vi "ConnectSetVarAtt.vi"(7 "VI reference":refnum<vi>, 8 "error in (no error)":errorcluster, 10 "Terms[]":refnum<vi>[][](array[refnum])) -> (0 "error out":errorcluster)   [LabVIEW 2009, in "HGF_VisitorGenerator.lvlib"]
doc: "wire set variant attribute in visitors appendData2Variant.vi"
uses:
  HGF_VisitorGenerator.lvlib
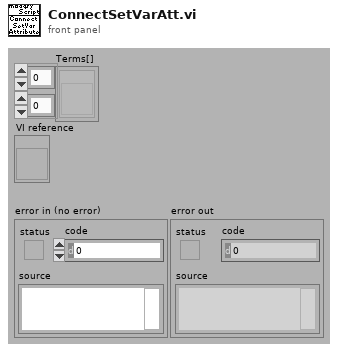
[diagram p1: front panel]
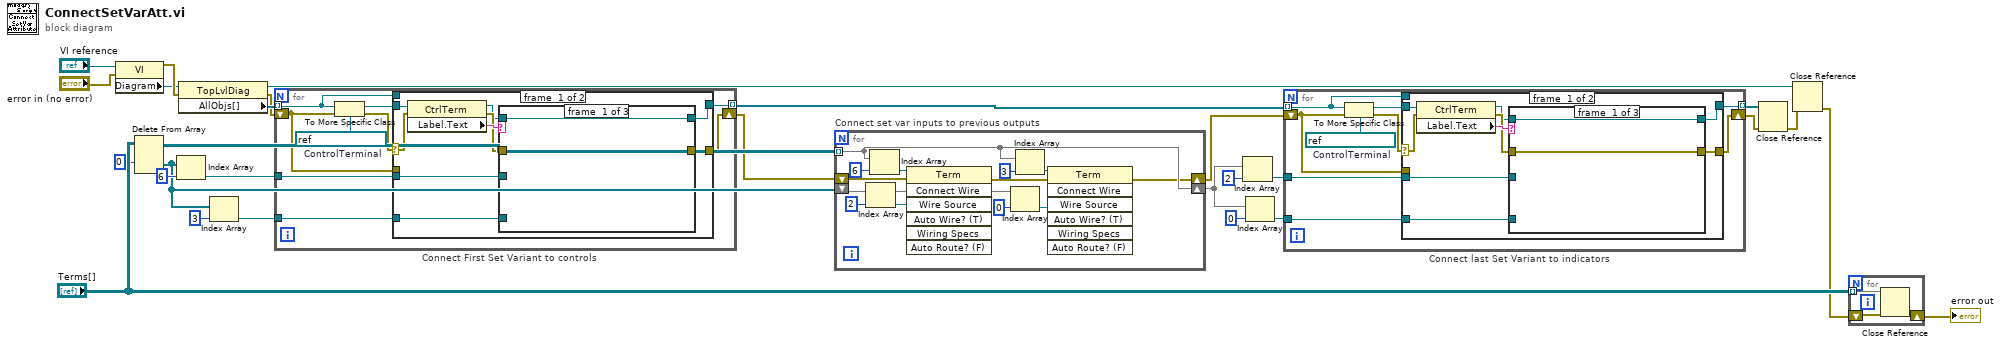
[diagram p0: block diagram]
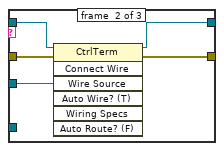
[diagram p2: hidden frame]
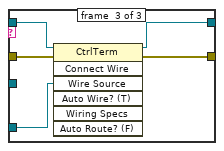
[diagram p3: hidden frame]
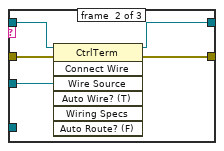
[diagram p5: hidden frame]
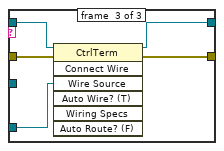
[diagram p6: hidden frame]
diagram:
  n1 = property class="VI"(reference="VI reference", error in="error in (no error)") -> (error out=w23:errorcluster, "Diagram"=w22:refnum<vi>)  [unwired: 1 out]
  n2 = Delete From Array(array="Terms[]", index (row)=0) -> (deleted portion=w13:refnum<vi>[], array with subset deleted=w14:refnum<vi>[][])  [unwired: 2 in]
  n3 = Index Array(array=w13, index=6) -> (element=w18:refnum<vi>)
  n4 = property class="TopLvlDiag"(reference=w22, error in=w23) -> (reference out=w21:refnum<vi>, error out=w17:errorcluster, "AllObjs[]"=w20:refnum<vi>[])
  n5 = Index Array(array=w13, index=3) -> (element=w15:refnum<vi>)
  n6 = for "Connect First Set Variant to controls" {
    tunnel: w20 -> [w31] mode=indexing
    tunnel: [w37] -> w10 mode=indexing
    tunnel: w18 -> [w30]
    shift-right: [w33] -> w12
    shift-left: w17 -> [w32]
    tunnel: w15 -> [w29]
    w35 = refnum<vi> refnum  # ControlTerminal
    n7 = To More Specific Class(target class=w35, reference=w31, error in=w32) -> (specific class reference=w36:refnum<vi>, error out=w34:errorcluster)
    n8 = case shown="No Error" w34 {
      selector: w34 -> [w45 _]
      tunnel: [w41 w59] -> w37
      tunnel: w36 -> [w46 _]
      tunnel: [w40 w60] -> w33
      tunnel: w32 -> [_ w60]
      tunnel: w31 -> [_ w59]
      tunnel: w30 -> [w39 _]
      tunnel: w29 -> [w38 _]
      frame #0 {
        n9 = property class="CtrlTerm"(reference=w46, error in=w45) -> (reference out=w42:refnum<vi>, error out=w43:errorcluster, "Label.Text"=w44:string)
        n10 = case shown="\"error in (no error)\"" w44 {
          tunnel: w43 -> [w47 w50 w55]
          tunnel: w42 -> [w48 w53 w58]
          tunnel: [w48 w52 w57] -> w41
          tunnel: [w47 w51 w56] -> w40
          tunnel: w39 -> [_ w49 _]
          tunnel: w38 -> [_ _ w54]
          frame #0 {
          }
          frame #1 {
            n11 = invoke class="CtrlTerm" method="Connect Wire"(reference=w53, error in=w50, "Wire Source"=w49) -> (reference out=w52:refnum<vi>, error out=w51:errorcluster)  [unwired: 4 in, 5 out]
          }
          frame #2 {
            n12 = invoke class="CtrlTerm" method="Connect Wire"(reference=w58, error in=w55, "Wire Source"=w54) -> (reference out=w57:refnum<vi>, error out=w56:errorcluster)  [unwired: 4 in, 5 out]
          }
        }
      }
      frame #1 {
      }
    }
  }
  n13 = for "Connect set var inputs to previous outputs" {
    tunnel: w14 -> [w68] mode=indexing
    shift-right: [w68] -> w4
    shift-left: w13 -> [w66]
    shift-right: [w61] -> w8
    shift-left: w12 -> [w63]
    n14 = Index Array(array=w66, index=2) -> (element=w70:refnum<vi>)
    n15 = Index Array(array=w68, index=6) -> (element=w72:refnum<vi>)
    n16 = invoke class="Term" method="Connect Wire"(reference=w72, error in=w63, "Wire Source"=w70) -> (error out=w62:errorcluster)  [unwired: 4 in, 6 out]
    n17 = Index Array(array=w66, index=0) -> (element=w64:refnum<vi>)
    n18 = Index Array(array=w68, index=3) -> (element=w69:refnum<vi>)
    n19 = invoke class="Term" method="Connect Wire"(reference=w69, error in=w62, "Wire Source"=w64) -> (error out=w61:errorcluster)  [unwired: 4 in, 6 out]
  }
  n20 = Index Array(array=w4, index=2) -> (element=w6:refnum<vi>)
  n21 = Index Array(array=w4, index=0) -> (element=w5:refnum<vi>)
  n22 = for "Connect last Set Variant to indicators" {
    tunnel: w10 -> [w76] mode=indexing
    tunnel: [w82] -> w9 mode=indexing
    tunnel: w6 -> [w75]
    shift-right: [w78] -> w7
    shift-left: w8 -> [w77]
    tunnel: w5 -> [w74]
    w80 = refnum<vi> refnum  # ControlTerminal
    n23 = To More Specific Class(target class=w80, reference=w76, error in=w77) -> (specific class reference=w81:refnum<vi>, error out=w79:errorcluster)
    n24 = case shown="No Error" w79 {
      selector: w79 -> [w90 _]
      tunnel: [w86 w104] -> w82
      tunnel: w81 -> [w91 _]
      tunnel: [w85 w105] -> w78
      tunnel: w77 -> [_ w105]
      tunnel: w76 -> [_ w104]
      tunnel: w75 -> [w84 _]
      tunnel: w74 -> [w83 _]
      frame #0 {
        n25 = property class="CtrlTerm"(reference=w91, error in=w90) -> (reference out=w87:refnum<vi>, error out=w88:errorcluster, "Label.Text"=w89:string)
        n26 = case shown="\"dup initData\"" w89 {
          tunnel: w88 -> [w92 w95 w100]
          tunnel: w87 -> [w93 w98 w103]
          tunnel: [w93 w97 w102] -> w86
          tunnel: [w92 w96 w101] -> w85
          tunnel: w84 -> [_ w94 _]
          tunnel: w83 -> [_ _ w99]
          frame #0 {
          }
          frame #1 {
            n27 = invoke class="CtrlTerm" method="Connect Wire"(reference=w98, error in=w95, "Wire Source"=w94) -> (reference out=w97:refnum<vi>, error out=w96:errorcluster)  [unwired: 4 in, 5 out]
          }
          frame #2 {
            n28 = invoke class="CtrlTerm" method="Connect Wire"(reference=w103, error in=w100, "Wire Source"=w99) -> (reference out=w102:refnum<vi>, error out=w101:errorcluster)  [unwired: 4 in, 5 out]
          }
        }
      }
      frame #1 {
      }
    }
  }
  n29 = Close Reference(reference=w9, error in (no error)=w7) -> (error out=w19:errorcluster)
  n30 = Close Reference(reference=w21, error in (no error)=w19) -> (error out=w1:errorcluster)
  n31 = for {
    tunnel: "Terms[]" -> [w108] mode=indexing
    shift-right: [w107] -> w28
    shift-left: w1 -> [w106]
    n32 = Close Reference(reference=w108, error in (no error)=w106) -> (error out=w107:errorcluster)
  }
  "error out" <- w28
